vi "Catch POP Errors.vi"(1 "error in":errorcluster, 2 "POP server response":string, 3 "Caller Path":path) -> (0 "error out":errorcluster)   [LabVIEW 2012]
doc: "This is a special-purpose error-handler VI used in the low-level POP command VIs.\n\nThis VI reserves an error code of 6000 to indicate that the mail server returned its error string (\"-ERR...\") in response to a low-level POP command, indicating that the POP command was invalid or that there were insufficient or improper arguments."
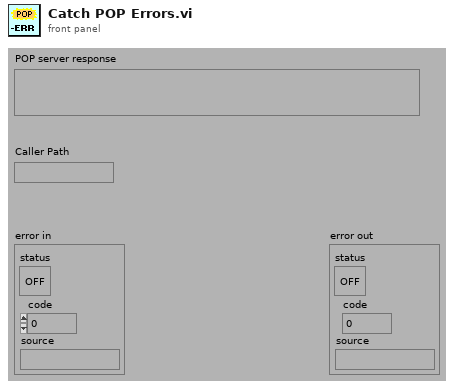
[diagram p1: front panel]
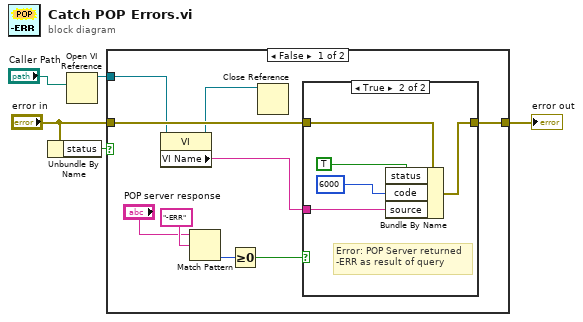
[diagram p0: block diagram]
diagram:
  n1 = Unbundle By Name("error in") -> ("status"=w4:bool)
  n2 = Open VI Reference(vi path="Caller Path") -> (vi reference=w1:refnum<vi>)  [unwired: 5 in, 1 out]
  n3 = case shown="False" w4 {
    tunnel: "error in" -> [w10 w21]
    tunnel: [w9 w21] -> w3
    tunnel: w1 -> [w7 _]
    frame False {
      n4 = property class="VI"(reference=w7) -> (reference out=w6:refnum<vi>, "VI Name"=w8:string)  [unwired: 1 in, 1 out]
      n5 = Match Pattern(string="POP server response", regular expression="-ERR") -> (offset past match=w14:i32)  [unwired: 1 in, 3 out]
      n6 = Greater Or Equal To 0?(x=w14) -> (x >= 0?=w11:bool)
      n7 = Close Reference(reference=w6) -> ()  [unwired: 1 in, 1 out]
      n8 = case shown="True" w11 {
        tunnel: w10 -> [w15 w20]
        tunnel: [w15 w17] -> w9
        tunnel: w8 -> [_ w16]
        frame False {
        }
        frame True {
          # "Error: POP Server returned\n-ERR as result of query"
          n9 = Bundle By Name(cluster=w20, "status"=TRUE, "code"=6000, "source"=w16) -> (w17:errorcluster)
        }
      }
    }
    frame True {
    }
  }
  "error out" <- w3
